vi "End BidirectionalStreamTemplate.vi"(8 "error in":errorcluster, 11 "Call ID in":T2) -> (0 "error out":errorcluster, 1 "errorDetails":T1)   [LabVIEW 2020, in "MeasurementLink Session Management Client.lvlib"]
uses:
  <vilib>/gRPC/LabVIEW gRPC Library/Shared/grpcId.ctl
  <vilib>/gRPC/LabVIEW gRPC Library/Shared/Any.ctl
  MeasurementLink Session Management Client.lvlib
  <vilib>/gRPC/LabVIEW gRPC Library/grpc-lvsupport-release.lvlib
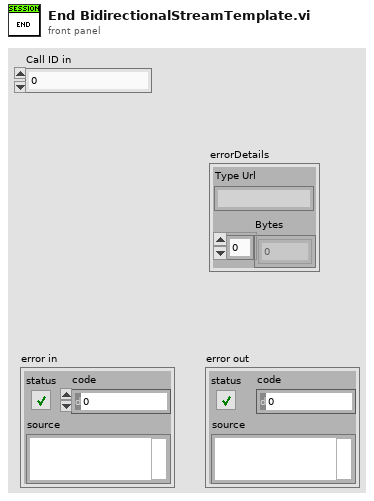
[diagram p1: front panel]
types:
  T1 = typedef "grpc-lvsupport-release.lvlib/Any.ctl" = cluster{"Type Url":string, "Bytes":u8[]}
  T2 = typedef "grpc-lvsupport-release.lvlib/grpcId.ctl" = u64
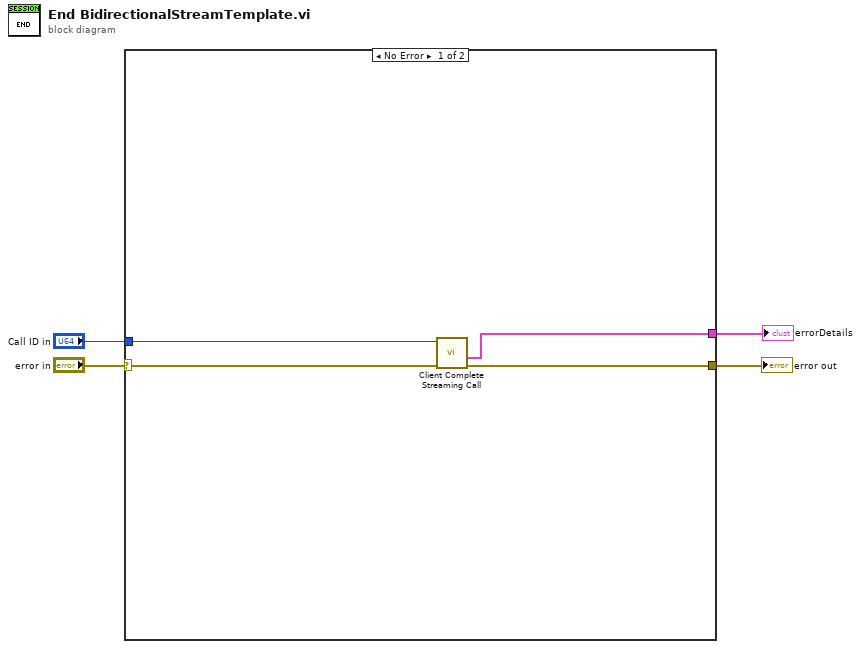
[diagram p0: block diagram]
diagram:
  n1 = case shown="No Error" "error in" {
    selector: "error in" -> [w7 w9]
    tunnel: [w6 w9] -> w3
    tunnel: "Call ID in" -> [w8 _]
    tunnel: [w5 _] -> w1
    frame No Error {
      n2 = call <vilib>:"Client Complete Streaming Call.vi"("error in"=w7, "Call ID in"=w8) -> ("error out"=w6:errorcluster, "errorDetails"=w5:T1)  [unwired: 8 in]
    }
    frame Error {
    }
  }
  "error out" <- w3
  "errorDetails" <- w1
